vi "Verify Set and Get Accessors for DSF Configuration.vi"(6 ".NET Refnum":refnum<k24>, 8 "error in":errorcluster, 10 "version":cluster{"major":u32, "minor":u32, "update":u32}={"major"=1, "minor"=0, "update"=0}, 11 "Set and Get Config Options Test in":refnum<class "Set and Get Config Options Test.lvclass">) -> (0 "error out":errorcluster, 3 "Set and Get Config Options Test out":refnum<class "Set and Get Config Options Test.lvclass">)   [LabVIEW 2017, in "Set and Get Config Options Test.lvclass"]
uses:
  Set and Get Config Options Test.lvclass
  NationalInstruments.VeriStand.SystemDefinitionAPI
  Scripting API/Data Sharing Framework Custom Device Scripting.lvlib
  Shared/DSF Shared.lvlib
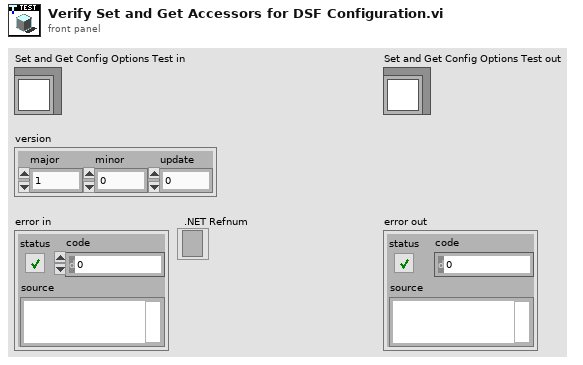
[diagram p1: front panel]
types:
  T1 = typedef "Custom Device API.lvlib/Custom Device Item Ref.ctl" = u64
  T2 = typedef "DSF Core.lvlibp/Framework.lvclass/Framework Options.ctl" = cluster{"FIFO Options":T3, "Thread Options":T4, "Plugin Options":T5, "Performance Options":T6, "Data Server Options":T7}
  T3 = typedef "DSF Core.lvlibp/Framework.lvclass/DSF FIFO Options.ctl" = cluster{"Infinite Timeouts":bool}
  T4 = typedef "DSF Core.lvlibp/Thread.lvclass/Thread Options.ctl" = cluster{"Show FP On Call":bool, "Close FP After Call":bool, "Allow Debugging":bool}
  T5 = typedef "DSF Core.lvlibp/Framework.lvclass/DSF Plugin Options.ctl" = cluster{"Default Components":bool}
  T6 = typedef "DSF Core.lvlibp/DSF Performance Options.ctl" = cluster{"Measure Period":bool, "Measure Rx/Tx Duration":bool}
  T7 = typedef "DSF Core.lvlibp/Framework.lvclass/Data Server Options.ctl" = cluster{"Enable Data Server":bool, "Period":u32}
  T8 = cluster{"measure period?":bool, "measure Rx/Tx duration?":bool}
  T9 = cluster{"enable data server":bool, "data server frequency (Hz)":dbl, "enable data server":bool}
  T10 = cluster{"data server enabled?":bool, "data server frequency (Hz)":dbl, "launch data viewer?":bool}
  T11 = cluster{"debug?":bool, "infinite FIFO timeouts?":bool}
  T12 = cluster{"show error dialog":bool, "show error dialog":bool}
  T13 = cluster{"show error dialog?":bool, "show threads?":bool}
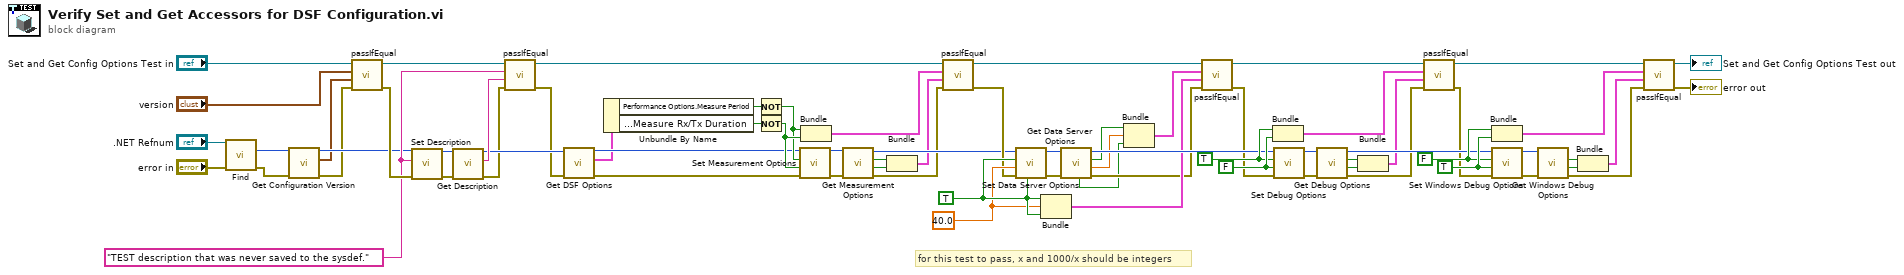
[diagram p0: block diagram]
diagram:
  w65 = TRUE ("show error dialog")
  w64 = FALSE ("show error dialog")
  w52 = FALSE ("debug")
  w51 = TRUE ("debug")
  w38 = 40.0 ("data server frequency (Hz)")
  w39 = TRUE ("enable data server")
  w12 = "TEST description that was never saved to the sysdef." ("description")
  # "for this test to pass, x and 1000/x should be integers"
  n1 = call "Find.vi"("error in"="error in", "target in"=".NET Refnum") -> ("error out"=w5:errorcluster, "data sharing framework custom device"=w4:T1)  [unwired: 7 in, 1 out]
  n2 = call "Get Configuration Version.vi"("error in"=w5, "data sharing framework custom device in"=w4) -> ("error out"=w8:errorcluster, "version"=w7:cluster{"major":u32, "minor":u32, "update":u32}, "data sharing framework custom device out"=w9:T1)  [unwired: 6 in, 1 out]
  n3 = call-dynamic "passIfEqual.vi"("error in (no error)"=w8, "y"=w7, "x"="version", "TestCase in"="Set and Get Config Options Test in") -> ("error out"=w13:errorcluster, "TestCase out"=w11:refnum<class "Set and Get Config Options Test.lvclass">)  [unwired: 6 in]
  n4 = call "Set Description.vi"("error in"=w13, "description"=w12, "data sharing framework custom device in"=w9) -> ("error out"=w14:errorcluster, "data sharing framework custom deviceout"=w10:T1)  [unwired: 7 in]
  n5 = call "Get Description.vi"("error in"=w14, "data sharing framework custom device in"=w10) -> ("error out"=w15:errorcluster, "description"=w18:string, "data sharing framework custom deviceout"=w17:T1)  [unwired: 7 in]
  n6 = call-dynamic "passIfEqual.vi"("error in (no error)"=w15, "y"=w18, "x"=w12, "TestCase in"=w11) -> ("error out"=w16:errorcluster, "TestCase out"=w33:refnum<class "Set and Get Config Options Test.lvclass">)  [unwired: 6 in]
  n7 = call "Get DSF Options.vi"("error in (no error)"=w16, "Item Ref in"=w17) -> ("error out"=w23:errorcluster, "options"=w19:T2, "Item Ref out"=w22:T1)  [unwired: 7 in]
  n8 = Unbundle By Name(w19) -> ("Performance Options.Measure Period"=w20:bool, "Performance Options.Measure Rx/Tx Duration"=w21:bool)
  n9 = Not(x=w20) -> (.not. x?=w26:bool)
  n10 = Not(x=w21) -> (.not. x?=w27:bool)
  n11 = call "Set Measurement Options.vi"("error in"=w23, "measure Rx/Tx duration"=w27, "measure period"=w26, "data sharing framework custom device in"=w22) -> ("error out"=w25:errorcluster, "data sharing framework custom device out"=w24:T1)  [unwired: 6 in]
  n12 = Bundle(w26, w27) -> (w31:cluster{bool, bool})  [unwired: 1 in]
  n13 = call "Get Measurement Options.vi"("error in"=w25, "data sharing framework custom device in"=w24) -> ("error out"=w32:errorcluster, "measure Rx/Tx duration?"=w29:bool, "measure period?"=w28:bool, "data sharing framework custom device out"=w34:T1)  [unwired: 6 in]
  n14 = Bundle("measure period?"=w28, "measure Rx/Tx duration?"=w29) -> (w30:T8)  [unwired: 1 in]
  n15 = call-dynamic "passIfEqual.vi"("error in (no error)"=w32, "y"=w30, "x"=w31, "TestCase in"=w33) -> ("error out"=w36:errorcluster, "TestCase out"=w43:refnum<class "Set and Get Config Options Test.lvclass">)  [unwired: 6 in]
  n16 = call "Set Data Server Options.vi"("launch data viewer"=w39, "error in"=w36, "data server frequency (Hz)"=w38, "enable data server"=w39, "data sharing framework custom device in"=w34) -> ("error out"=w37:errorcluster, "data sharing framework custom device out"=w35:T1)  [unwired: 5 in]
  n17 = Bundle("enable data server"=w39, "data server frequency (Hz)"=w38, "enable data server"=w39) -> (w45:T9)  [unwired: 1 in]
  n18 = call "Get Data Server Options.vi"("error in"=w37, "data sharing framework custom device in"=w35) -> ("error out"=w44:errorcluster, "data server frequency (Hz)"=w41:dbl, "data server enabled?"=w40:bool, "data sharing framework custom device out"=w48:T1, "launch data viewer?"=w42:bool)  [unwired: 5 in]
  n19 = Bundle("data server enabled?"=w40, "data server frequency (Hz)"=w41, "launch data viewer?"=w42) -> (w46:T10)  [unwired: 1 in]
  n20 = call-dynamic "passIfEqual.vi"("error in (no error)"=w44, "y"=w45, "x"=w46, "TestCase in"=w43) -> ("error out"=w47:errorcluster, "TestCase out"=w56:refnum<class "Set and Get Config Options Test.lvclass">)  [unwired: 6 in]
  n21 = Bundle("debug"=w51, "debug"=w52) -> (w57:cluster{"debug":bool, "debug":bool})  [unwired: 1 in]
  n22 = call "Set Debug Options.vi"("error in"=w47, "infinite FIFO timeouts"=w52, "debug"=w51, "data sharing framework custom device in"=w48) -> ("error out"=w49:errorcluster, "data sharing framework custom device out"=w50:T1)  [unwired: 6 in]
  n23 = call "Get Debug Options.vi"("error in"=w49, "data sharing framework custom device in"=w50) -> ("error out"=w55:errorcluster, "infinite FIFO timeouts?"=w54:bool, "debug?"=w53:bool, "data sharing framework custom device out"=w62:T1)  [unwired: 6 in]
  n24 = Bundle("debug?"=w53, "infinite FIFO timeouts?"=w54) -> (w58:T11)  [unwired: 1 in]
  n25 = call-dynamic "passIfEqual.vi"("error in (no error)"=w55, "y"=w58, "x"=w57, "TestCase in"=w56) -> ("error out"=w61:errorcluster, "TestCase out"=w67:refnum<class "Set and Get Config Options Test.lvclass">)  [unwired: 6 in]
  n26 = Bundle("show error dialog"=w64, "show error dialog"=w65) -> (w60:T12)  [unwired: 1 in]
  n27 = call "Set Windows Debug Options.vi"("error in"=w61, "show threads"=w65, "show error dialog"=w64, "data sharing framework custom device in"=w62) -> ("error out"=w66:errorcluster, "data sharing framework custom device out"=w63:T1)  [unwired: 6 in]
  n28 = call "Get Windows Debug Options.vi"("error in"=w66, "data sharing framework custom device in"=w63) -> ("error out"=w70:errorcluster, "show threads?"=w69:bool, "show error dialog?"=w68:bool)  [unwired: 6 in, 1 out]
  n29 = Bundle("show error dialog?"=w68, "show threads?"=w69) -> (w59:T13)  [unwired: 1 in]
  n30 = call-dynamic "passIfEqual.vi"("error in (no error)"=w70, "y"=w59, "x"=w60, "TestCase in"=w67) -> ("error out"=→"error out":errorcluster, "TestCase out"=→"Set and Get Config Options Test out":refnum<class "Set and Get Config Options Test.lvclass">)  [unwired: 6 in]
